vi "Init.vi"(8 "Error In":errorcluster, 11 "Communicator in":refnum<class "Communicator.lvclass">) -> (0 "Error Out":errorcluster, 3 "Communicator out":refnum<class "Communicator.lvclass">)   [LabVIEW 2024, in "Communicator.lvclass"]
uses:
  Communicator.lvclass
  Source/Interfaces/IConfigure/IConfigure.lvclass
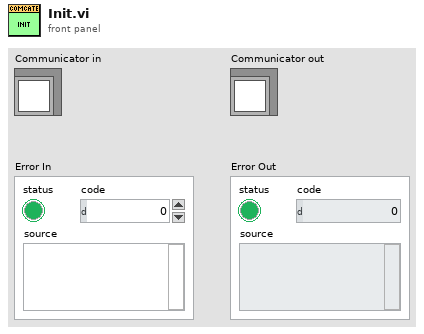
[diagram p1: front panel]
types:
  T1 = typedef "Communicator.lvclass/ObjectAttributes.ctl" = cluster{"IConfigure":refnum<class "IConfigure.lvclass">}
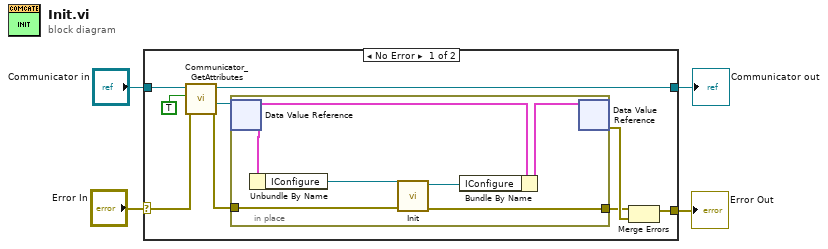
[diagram p0: block diagram]
diagram:
  n1 = case shown="No Error" "Error In" {
    selector: "Error In" -> [w12 w21]
    tunnel: [w9 w21] -> w3
    tunnel: [w10 w20] -> w1
    tunnel: "Communicator in" -> [w13 w20]
    frame No Error {
      n2 = call "Communicator_GetAttributes.vi"("Error In"=w12, "OnlyGetDvrReference(False)"=TRUE, "Communicator in"=w13) -> ("Error Out"=w6:errorcluster, "DataRef"=w8:refnum<data-value>, "Communicator out"=w10:refnum<class "Communicator.lvclass">)  [unwired: 5 in, 1 out]
      n3 = in-place {
        in-place-border: w6 -> [w17]
        in-place-border: [w14] -> w5
        n4 = in-place-dvr #1(w8) -> (w18:T1)  [unwired: 1 out]
        n5 = Unbundle By Name(w18) -> ("IConfigure"=w16:refnum<class "IConfigure.lvclass">)
        n6 = call-dynamic "Init.vi"("error in (no error)"=w17, "IConfigure in"=w16) -> ("error out"=w14:errorcluster, "IConfigure out"=w15:refnum<class "IConfigure.lvclass">)  [unwired: 8 in]
        n7 = Bundle By Name(cluster=w18, "IConfigure"=w15) -> (w19:T1)
        n8 = in-place-dvr #1(w19) -> (w11:errorcluster)  [unwired: 1 out]
      }
      n9 = Merge Errors(w5, w11) -> (w9:errorcluster)
    }
    frame Error {
    }
  }
  "Error Out" <- w3
  "Communicator out" <- w1
